vi "Get External Trigger Termination.vi"(11 "puiTermination":u32) -> (2 "function return":u32, 3 "puiTermination out":u32)   [LabVIEW 2018, in "AndorSDK.lvlib"]
doc: "EXPNETTYPE unsigned int WINAPI GetExternalTriggerTermination(at_u32 * puiTermination);"
uses:
  AndorSDK.lvlib
  ATMCD32D.dll
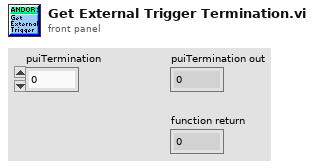
[diagram p1: front panel]
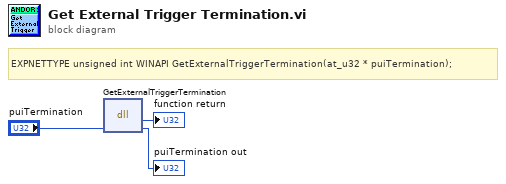
[diagram p0: block diagram]
diagram:
  # "EXPNETTYPE unsigned int WINAPI GetExternalTriggerTermination(at_u32 * puiTermination);"
  n1 = dll-call lib="PTH2babs E\nPersönliches02 - Arbeit03-HiwijobsLabviewCodelibANDOR\tAndor SDK\nATMCD32D.*" fn="GetExternalTriggerTermination"("puiTermination"="puiTermination") -> (→"function return":u32, "puiTermination"=→"puiTermination out":u32)  [unwired: 3 in, 2 out]
